vi "tsapp_transmit_flexray_async.vi"(7 "error in (no error)":errorcluster caption="错误输入（无错误）", 9 "FR_Transmit":T1={"FIdxChn"=0, "FChannelMask"=0, "FActualPayloadLength"=0, "FCycleNumber"=0, "FSlotId"=0, "Send_Array"=[1, 2, 3, 4, 5, 6, 7, 8, 9, 10, 11]} {"Send_Array" format="%.0x"}, 10 "Path":path) -> (0 "error out":errorcluster caption="错误输出", 2 "return":i32, 3 "Path output":path)   [LabVIEW 2014]
doc: "Function Introduction: Asynchronous Transmission of Flexray Messages\nCall location\nInput parameter AFlexray: flexray message pointer\nReturn value==0: Successful execution\nOther values: Query error code"
uses:
  Typedef/TLibFLexRay.ctl
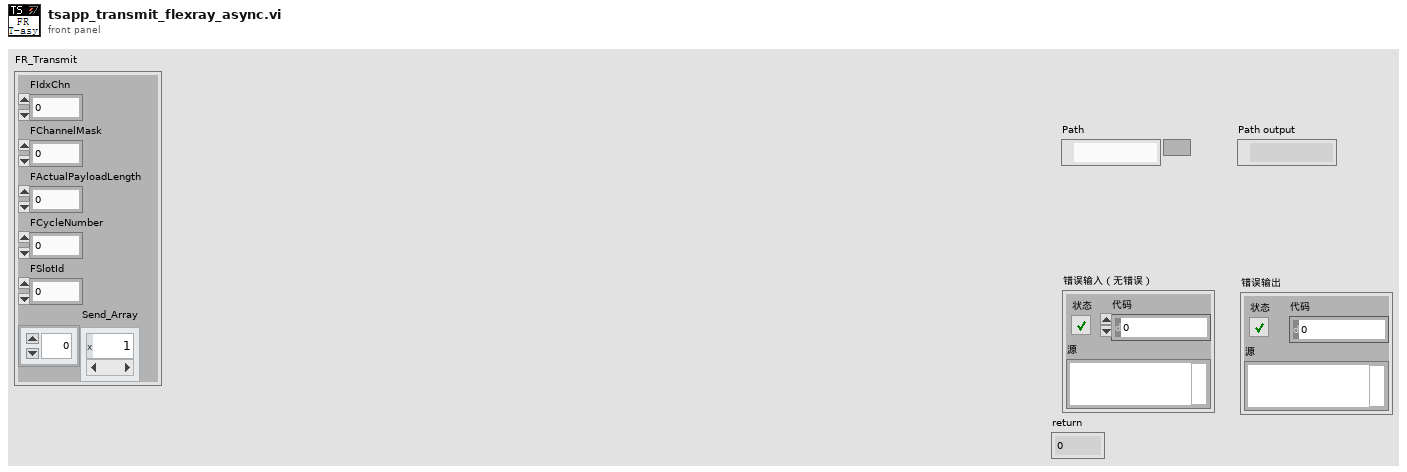
[diagram p1: front panel]
types:
  T1 = cluster{"FIdxChn":u8, "FChannelMask":u8, "FActualPayloadLength":u8, "FCycleNumber":u8, "FSlotId":u16, "Send_Array":u8[]}
  T2 = typedef "TLibFLexRay.ctl" = cluster{"FIdxChn":u8, "FChannelMask":u8, "FDir":u8, "FPayloadLength":u8, "FActualPayloadLength":u8, "FCycleNumber":u8, "FCCType":u8, "FFrameType":u8, "FHeaderCRCA":u16, "FHeaderCRCB":u16, "FFrameStateInfo":u16, "FSlotId":u16, "FFrameFlags":u32, "FFrameCRC":u32, "FReserved1":u64, "FReserved2":u64, "FTimeUs":u64, "FData":cluster{"数值":u8, "数值 9":u8, "数值 17":u8, "数值 25":u8, "数值 33":u8, "数值 41":u8, "数值 49":u8, "数值 57":u8, "数值 65":u8, "数值 73":u8, "数值 81":u8, "数值 89":u8, "数值 97":u8, "数值 105":u8, "数值 98":u8, "数值 99":u8, "数值 2":u8, "数值 10":u8, "数值 18":u8, "数值 26":u8, "数值 34":u8, "数值 42":u8, "数值 50":u8, "数值 58":u8, "数值 66":u8, "数值 74":u8, "数值 82":u8, "数值 90":u8, "数值 100":u8, "数值 106":u8, "数值 101":u8, "数值 102":u8, "数值 3":u8, "数值 11":u8, "数值 19":u8, "数值 27":u8, "数值 35":u8, "数值 43":u8, "数值 51":u8, "数值 59":u8, "数值 67":u8, "数值 75":u8, "数值 83":u8, "数值 91":u8, "数值 103":u8, "数值 107":u8, "数值 104":u8, "数值 108":u8, "数值 4":u8, "数值 12":u8, "数值 20":u8, "数值 28":u8, "数值 36":u8, "数值 44":u8, "数值 52":u8, "数值 60":u8, "数值 68":u8, "数值 76":u8, "数值 84":u8, "数值 92":u8, "数值 109":u8, "数值 110":u8, "数值 111":u8, "数值 112":u8, "数值 5":u8, "数值 13":u8, "数值 21":u8, "数值 29":u8, "数值 37":u8, "数值 45":u8, "数值 53":u8, "数值 61":u8, "数值 69":u8, "数值 77":u8, "数值 85":u8, "数值 93":u8, "数值 113":u8, "数值 114":u8, "数值 115":u8, "数值 116":u8, "数值 6":u8, "数值 14":u8, "数值 22":u8, "数值 30":u8, "数值 38":u8, "数值 46":u8, "数值 54":u8, "数值 62":u8, "数值 70":u8, "数值 78":u8, "数值 86":u8, "数值 94":u8, "数值 117":u8, "数值 118":u8, "数值 119":u8, "数值 120":u8, "数值 7":u8, "数值 15":u8, "数值 23":u8, "数值 31":u8, "数值 39":u8, "数值 47":u8, "数值 55":u8, "数值 63":u8, "数值 71":u8, "数值 79":u8, "数值 87":u8, "数值 95":u8, "数值 121":u8, "数值 122":u8, "数值 123":u8, "数值 124":u8, "数值 8":u8, "数值 16":u8, "数值 24":u8, "数值 32":u8, "数值 40":u8, "数值 48":u8, "数值 56":u8, "数值 64":u8, "数值 72":u8, "数值 80":u8, "数值 88":u8, "数值 96":u8, "数值 125":u8, "数值 126":u8, "数值 127":u8, "数值 128":u8, "数值 129":u8, "数值 130":u8, "数值 131":u8, "数值 132":u8, "数值 133":u8, "数值 134":u8, "数值 135":u8, "数值 136":u8, "数值 137":u8, "数值 138":u8, "数值 139":u8, "数值 140":u8, "数值 141":u8, "数值 142":u8, "数值 143":u8, "数值 144":u8, "数值 145":u8, "数值 146":u8, "数值 147":u8, "数值 148":u8, "数值 149":u8, "数值 150":u8, "数值 151":u8, "数值 152":u8, "数值 153":u8, "数值 154":u8, "数值 155":u8, "数值 156":u8, "数值 157":u8, "数值 158":u8, "数值 159":u8, "数值 160":u8, "数值 161":u8, "数值 162":u8, "数值 163":u8, "数值 164":u8, "数值 165":u8, "数值 166":u8, "数值 167":u8, "数值 168":u8, "数值 169":u8, "数值 170":u8, "数值 171":u8, "数值 172":u8, "数值 173":u8, "数值 174":u8, "数值 175":u8, "数值 176":u8, "数值 177":u8, "数值 178":u8, "数值 179":u8, "数值 180":u8, "数值 181":u8, "数值 182":u8, "数值 183":u8, "数值 184":u8, "数值 185":u8, "数值 186":u8, "数值 187":u8, "数值 188":u8, "数值 189":u8, "数值 190":u8, "数值 191":u8, "数值 192":u8, "数值 193":u8, "数值 194":u8, "数值 195":u8, "数值 196":u8, "数值 197":u8, "数值 198":u8, "数值 199":u8, "数值 200":u8, "数值 201":u8, "数值 202":u8, "数值 203":u8, "数值 204":u8, "数值 205":u8, "数值 206":u8, "数值 207":u8, "数值 208":u8, "数值 209":u8, "数值 210":u8, "数值 211":u8, "数值 212":u8, "数值 213":u8, "数值 214":u8, "数值 215":u8, "数值 216":u8, "数值 217":u8, "数值 218":u8, "数值 219":u8, "数值 220":u8, "数值 221":u8, "数值 222":u8, "数值 223":u8, "数值 224":u8, "数值 225":u8, "数值 226":u8, "数值 227":u8, "数值 228":u8, "数值 229":u8, "数值 230":u8, "数值 231":u8, "数值 232":u8, "数值 233":u8, "数值 234":u8, "数值 235":u8, "数值 236":u8, "数值 237":u8, "数值 238":u8, "数值 239":u8, "数值 241":u8, "数值 242":u8, "数值 243":u8, "数值 244":u8, "数值 245":u8, "数值 246":u8, "数值 247":u8, "数值 248":u8, "数值 249":u8, "数值 250":u8, "数值 251":u8, "数值 252":u8, "数值 253":u8, "数值 254":u8, "数值 255":u8}}
  T3 = cluster{"Send_Array[0]":u8, "Send_Array[1]":u8, "Send_Array[2]":u8, "Send_Array[3]":u8, "Send_Array[4]":u8, "Send_Array[5]":u8, "Send_Array[6]":u8, "Send_Array[7]":u8, "Send_Array[8]":u8, "Send_Array[9]":u8, "Send_Array[10]":u8, "Send_Array[11]":u8, "Send_Array[12]":u8, "Send_Array[13]":u8, "Send_Array[14]":u8, "Send_Array[15]":u8, "Send_Array[16]":u8, "Send_Array[17]":u8, "Send_Array[18]":u8, "Send_Array[19]":u8, "Send_Array[20]":u8, "Send_Array[21]":u8, "Send_Array[22]":u8, "Send_Array[23]":u8, "Send_Array[24]":u8, "Send_Array[25]":u8, "Send_Array[26]":u8, "Send_Array[27]":u8, "Send_Array[28]":u8, "Send_Array[29]":u8, "Send_Array[30]":u8, "Send_Array[31]":u8, "Send_Array[32]":u8, "Send_Array[33]":u8, "Send_Array[34]":u8, "Send_Array[35]":u8, "Send_Array[36]":u8, "Send_Array[37]":u8, "Send_Array[38]":u8, "Send_Array[39]":u8, "Send_Array[40]":u8, "Send_Array[41]":u8, "Send_Array[42]":u8, "Send_Array[43]":u8, "Send_Array[44]":u8, "Send_Array[45]":u8, "Send_Array[46]":u8, "Send_Array[47]":u8, "Send_Array[48]":u8, "Send_Array[49]":u8, "Send_Array[50]":u8, "Send_Array[51]":u8, "Send_Array[52]":u8, "Send_Array[53]":u8, "Send_Array[54]":u8, "Send_Array[55]":u8, "Send_Array[56]":u8, "Send_Array[57]":u8, "Send_Array[58]":u8, "Send_Array[59]":u8, "Send_Array[60]":u8, "Send_Array[61]":u8, "Send_Array[62]":u8, "Send_Array[63]":u8, "Send_Array[64]":u8, "Send_Array[65]":u8, "Send_Array[66]":u8, "Send_Array[67]":u8, "Send_Array[68]":u8, "Send_Array[69]":u8, "Send_Array[70]":u8, "Send_Array[71]":u8, "Send_Array[72]":u8, "Send_Array[73]":u8, "Send_Array[74]":u8, "Send_Array[75]":u8, "Send_Array[76]":u8, "Send_Array[77]":u8, "Send_Array[78]":u8, "Send_Array[79]":u8, "Send_Array[80]":u8, "Send_Array[81]":u8, "Send_Array[82]":u8, "Send_Array[83]":u8, "Send_Array[84]":u8, "Send_Array[85]":u8, "Send_Array[86]":u8, "Send_Array[87]":u8, "Send_Array[88]":u8, "Send_Array[89]":u8, "Send_Array[90]":u8, "Send_Array[91]":u8, "Send_Array[92]":u8, "Send_Array[93]":u8, "Send_Array[94]":u8, "Send_Array[95]":u8, "Send_Array[96]":u8, "Send_Array[97]":u8, "Send_Array[98]":u8, "Send_Array[99]":u8, "Send_Array[100]":u8, "Send_Array[101]":u8, "Send_Array[102]":u8, "Send_Array[103]":u8, "Send_Array[104]":u8, "Send_Array[105]":u8, "Send_Array[106]":u8, "Send_Array[107]":u8, "Send_Array[108]":u8, "Send_Array[109]":u8, "Send_Array[110]":u8, "Send_Array[111]":u8, "Send_Array[112]":u8, "Send_Array[113]":u8, "Send_Array[114]":u8, "Send_Array[115]":u8, "Send_Array[116]":u8, "Send_Array[117]":u8, "Send_Array[118]":u8, "Send_Array[119]":u8, "Send_Array[120]":u8, "Send_Array[121]":u8, "Send_Array[122]":u8, "Send_Array[123]":u8, "Send_Array[124]":u8, "Send_Array[125]":u8, "Send_Array[126]":u8, "Send_Array[127]":u8, "Send_Array[128]":u8, "Send_Array[129]":u8, "Send_Array[130]":u8, "Send_Array[131]":u8, "Send_Array[132]":u8, "Send_Array[133]":u8, "Send_Array[134]":u8, "Send_Array[135]":u8, "Send_Array[136]":u8, "Send_Array[137]":u8, "Send_Array[138]":u8, "Send_Array[139]":u8, "Send_Array[140]":u8, "Send_Array[141]":u8, "Send_Array[142]":u8, "Send_Array[143]":u8, "Send_Array[144]":u8, "Send_Array[145]":u8, "Send_Array[146]":u8, "Send_Array[147]":u8, "Send_Array[148]":u8, "Send_Array[149]":u8, "Send_Array[150]":u8, "Send_Array[151]":u8, "Send_Array[152]":u8, "Send_Array[153]":u8, "Send_Array[154]":u8, "Send_Array[155]":u8, "Send_Array[156]":u8, "Send_Array[157]":u8, "Send_Array[158]":u8, "Send_Array[159]":u8, "Send_Array[160]":u8, "Send_Array[161]":u8, "Send_Array[162]":u8, "Send_Array[163]":u8, "Send_Array[164]":u8, "Send_Array[165]":u8, "Send_Array[166]":u8, "Send_Array[167]":u8, "Send_Array[168]":u8, "Send_Array[169]":u8, "Send_Array[170]":u8, "Send_Array[171]":u8, "Send_Array[172]":u8, "Send_Array[173]":u8, "Send_Array[174]":u8, "Send_Array[175]":u8, "Send_Array[176]":u8, "Send_Array[177]":u8, "Send_Array[178]":u8, "Send_Array[179]":u8, "Send_Array[180]":u8, "Send_Array[181]":u8, "Send_Array[182]":u8, "Send_Array[183]":u8, "Send_Array[184]":u8, "Send_Array[185]":u8, "Send_Array[186]":u8, "Send_Array[187]":u8, "Send_Array[188]":u8, "Send_Array[189]":u8, "Send_Array[190]":u8, "Send_Array[191]":u8, "Send_Array[192]":u8, "Send_Array[193]":u8, "Send_Array[194]":u8, "Send_Array[195]":u8, "Send_Array[196]":u8, "Send_Array[197]":u8, "Send_Array[198]":u8, "Send_Array[199]":u8, "Send_Array[200]":u8, "Send_Array[201]":u8, "Send_Array[202]":u8, "Send_Array[203]":u8, "Send_Array[204]":u8, "Send_Array[205]":u8, "Send_Array[206]":u8, "Send_Array[207]":u8, "Send_Array[208]":u8, "Send_Array[209]":u8, "Send_Array[210]":u8, "Send_Array[211]":u8, "Send_Array[212]":u8, "Send_Array[213]":u8, "Send_Array[214]":u8, "Send_Array[215]":u8, "Send_Array[216]":u8, "Send_Array[217]":u8, "Send_Array[218]":u8, "Send_Array[219]":u8, "Send_Array[220]":u8, "Send_Array[221]":u8, "Send_Array[222]":u8, "Send_Array[223]":u8, "Send_Array[224]":u8, "Send_Array[225]":u8, "Send_Array[226]":u8, "Send_Array[227]":u8, "Send_Array[228]":u8, "Send_Array[229]":u8, "Send_Array[230]":u8, "Send_Array[231]":u8, "Send_Array[232]":u8, "Send_Array[233]":u8, "Send_Array[234]":u8, "Send_Array[235]":u8, "Send_Array[236]":u8, "Send_Array[237]":u8, "Send_Array[238]":u8, "Send_Array[239]":u8, "Send_Array[240]":u8, "Send_Array[241]":u8, "Send_Array[242]":u8, "Send_Array[243]":u8, "Send_Array[244]":u8, "Send_Array[245]":u8, "Send_Array[246]":u8, "Send_Array[247]":u8, "Send_Array[248]":u8, "Send_Array[249]":u8, "Send_Array[250]":u8, "Send_Array[251]":u8, "Send_Array[252]":u8, "Send_Array[253]":u8}
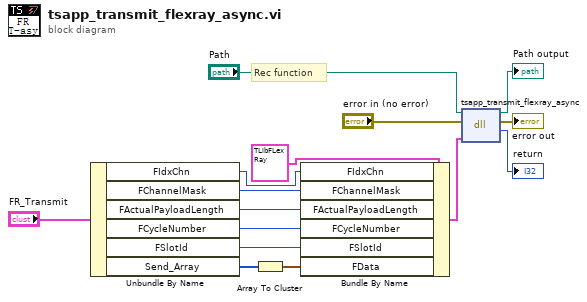
[diagram p0: block diagram]
diagram:
  # "Rec function"
  n1 = Unbundle By Name("FR_Transmit") -> ("FIdxChn"=w6:u8, "FChannelMask"=w5:u8, "FActualPayloadLength"=w4:u8, "FCycleNumber"=w3:u8, "FSlotId"=w2:u16, "Send_Array"=w7:u8[])
  n2 = Array To Cluster(array=w7) -> (cluster=w1:T3)
  n3 = Bundle By Name(cluster=T2 {"FIdxChn"=0, "FChannelMask"=0, "FDir"=0, "FPayloadLength"=0, "FActualPayloadLength"=0, "FCycleNumber"=0, "FCCType"=0, "FFrameType"=0, "FHeaderCRCA"=0, "FHeaderCRCB"=0, "FFrameStateInfo"=0, "FSlotId"=0, "FFrameFlags"=0, "FFrameCRC"=0, "FReserved1"=0, "FReserved2"=0, "FTimeUs"=0, "FData"={"数值"=0, "数值 9"=0, "数值 17"=0, "数值 25"=0, "数值 33"=0, "数值 41"=0, "数值 49"=0, "数值 57"=0, "数值 65"=0, "数值 73"=0, "数值 81"=0, "数值 89"=0, "数值 97"=0, "数值 105"=0, "数值 98"=0, "数值 99"=0, "数值 2"=0, "数值 10"=0, "数值 18"=0, "数值 26"=0, "数值 34"=0, "数值 42"=0, "数值 50"=0, "数值 58"=0, "数值 66"=0, "数值 74"=0, "数值 82"=0, "数值 90"=0, "数值 100"=0, "数值 106"=0, "数值 101"=0, "数值 102"=0, "数值 3"=0, "数值 11"=0, "数值 19"=0, "数值 27"=0, "数值 35"=0, "数值 43"=0, "数值 51"=0, "数值 59"=0, "数值 67"=0, "数值 75"=0, "数值 83"=0, "数值 91"=0, "数值 103"=0, "数值 107"=0, "数值 104"=0, "数值 108"=0, "数值 4"=0, "数值 12"=0, "数值 20"=0, "数值 28"=0, "数值 36"=0, "数值 44"=0, "数值 52"=0, "数值 60"=0, "数值 68"=0, "数值 76"=0, "数值 84"=0, "数值 92"=0, "数值 109"=0, "数值 110"=0, "数值 111"=0, "数值 112"=0, "数值 5"=0, "数值 13"=0, "数值 21"=0, "数值 29"=0, "数值 37"=0, "数值 45"=0, "数值 53"=0, "数值 61"=0, "数值 69"=0, "数值 77"=0, "数值 85"=0, "数值 93"=0, "数值 113"=0, "数值 114"=0, "数值 115"=0, "数值 116"=0, "数值 6"=0, "数值 14"=0, "数值 22"=0, "数值 30"=0, "数值 38"=0, "数值 46"=0, "数值 54"=0, "数值 62"=0, "数值 70"=0, "数值 78"=0, "数值 86"=0, "数值 94"=0, "数值 117"=0, "数值 118"=0, "数值 119"=0, "数值 120"=0, "数值 7"=0, "数值 15"=0, "数值 23"=0, "数值 31"=0, "数值 39"=0, "数值 47"=0, "数值 55"=0, "数值 63"=0, "数值 71"=0, "数值 79"=0, "数值 87"=0, "数值 95"=0, "数值 121"=0, "数值 122"=0, "数值 123"=0, "数值 124"=0, "数值 8"=0, "数值 16"=0, "数值 24"=0, "数值 32"=0, "数值 40"=0, "数值 48"=0, "数值 56"=0, "数值 64"=0, "数值 72"=0, "数值 80"=0, "数值 88"=0, "数值 96"=0, "数值 125"=0, "数值 126"=0, "数值 127"=0, "数值 128"=0, "数值 129"=0, "数值 130"=0, "数值 131"=0, "数值 132"=0, "数值 133"=0, "数值 134"=0, "数值 135"=0, "数值 136"=0, "数值 137"=0, "数值 138"=0, "数值 139"=0, "数值 140"=0, "数值 141"=0, "数值 142"=0, "数值 143"=0, "数值 144"=0, "数值 145"=0, "数值 146"=0, "数值 147"=0, "数值 148"=0, "数值 149"=0, "数值 150"=0, "数值 151"=0, "数值 152"=0, "数值 153"=0, "数值 154"=0, "数值 155"=0, "数值 156"=0, "数值 157"=0, "数值 158"=0, "数值 159"=0, "数值 160"=0, "数值 161"=0, "数值 162"=0, "数值 163"=0, "数值 164"=0, "数值 165"=0, "数值 166"=0, "数值 167"=0, "数值 168"=0, "数值 169"=0, "数值 170"=0, "数值 171"=0, "数值 172"=0, "数值 173"=0, "数值 174"=0, "数值 175"=0, "数值 176"=0, "数值 177"=0, "数值 178"=0, "数值 179"=0, "数值 180"=0, "数值 181"=0, "数值 182"=0, "数值 183"=0, "数值 184"=0, "数值 185"=0, "数值 186"=0, "数值 187"=0, "数值 188"=0, "数值 189"=0, "数值 190"=0, "数值 191"=0, "数值 192"=0, "数值 193"=0, "数值 194"=0, "数值 195"=0, "数值 196"=0, "数值 197"=0, "数值 198"=0, "数值 199"=0, "数值 200"=0, "数值 201"=0, "数值 202"=0, "数值 203"=0, "数值 204"=0, "数值 205"=0, "数值 206"=0, "数值 207"=0, "数值 208"=0, "数值 209"=0, "数值 210"=0, "数值 211"=0, "数值 212"=0, "数值 213"=0, "数值 214"=0, "数值 215"=0, "数值 216"=0, "数值 217"=0, "数值 218"=0, "数值 219"=0, "数值 220"=0, "数值 221"=0, "数值 222"=0, "数值 223"=0, "数值 224"=0, "数值 225"=0, "数值 226"=0, "数值 227"=0, "数值 228"=0, "数值 229"=0, "数值 230"=0, "数值 231"=0, "数值 232"=0, "数值 233"=0, "数值 234"=0, "数值 235"=0, "数值 236"=0, "数值 237"=0, "数值 238"=0, "数值 239"=0, "数值 241"=0, "数值 242"=0, "数值 243"=0, "数值 244"=0, "数值 245"=0, "数值 246"=0, "数值 247"=0, "数值 248"=0, "数值 249"=0, "数值 250"=0, "数值 251"=0, "数值 252"=0, "数值 253"=0, "数值 254"=0, "数值 255"=0}} ("TLibFLexRay"), "FIdxChn"=w6, "FChannelMask"=w5, "FActualPayloadLength"=w4, "FCycleNumber"=w3, "FSlotId"=w2, "FData"=w1) -> (w9:T2)
  n4 = dll-call lib="D:/Program Files (x86)/TOSUN/TSMaster/bin64/TSMaster.dll" fn="tsapp_transmit_flexray_async"(path in="Path", error in="error in (no error)", "AFlexRay"=w9) -> (path out=→"Path output":path, error out=→"error out":errorcluster, "return"=→"return":i32)  [unwired: 2 in]
